vi "(SubVI)Scope_Log_Write Header.vi"(8 "에러 입력(에러 없음)":errorcluster, 10 "Scope_Channel Settings":T1[](array[typedef]) {"Address" format="%04x"}, 11 "Path":path) -> (0 "에러 출력":errorcluster, 3 "File Ref":refnum<file>)   [LabVIEW 2020]
uses:
  Controls/(Ctrl)Scope_Settings.ctl
  e063a442-55f0-4c5f-88aa-a2279cc821e3.vi
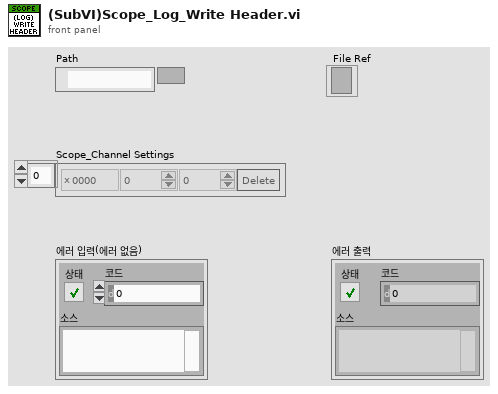
[diagram p1: front panel]
types:
  T1 = typedef "(Ctrl)Scope_Settings.ctl" = cluster{"Address":u16, "Scale":i32, "Offset":i32, "Delete":bool}
  T2 = enum16{"open", "replace", "create", "open or create", "replace or create", "replace or create with confirmation"}
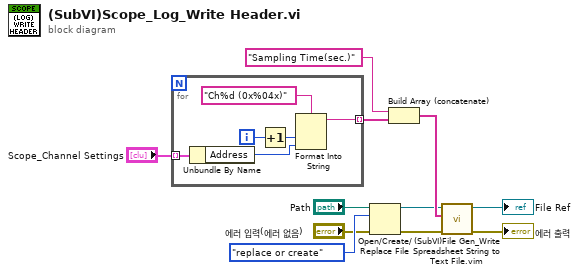
[diagram p0: block diagram]
diagram:
  n1 = for {
    tunnel: "Scope_Channel Settings" -> [w17] mode=indexing
    tunnel: [w12] -> w5 mode=indexing
    i -> [w16]
    n2 = Unbundle By Name(w17) -> ("Address"=w13:u16)
    n3 = Increment(x=w16) -> (x+1=w14:i32)
    n4 = Format Into String(format string="Ch%d (0x%04x)" ("포맷 문자열"), w14, w13) -> (resulting string=w12:string)  [unwired: 2 in, 1 out]
  }
  n5 = Open/Create/Replace File(file path (use dialog)="Path", error in="에러 입력(에러 없음)", operation (0:open)=T2."replace or create" ("동작(0:open)")) -> (refnum out=w7:refnum<file>, error out=w8:errorcluster)  [unwired: 3 in, 1 out]
  n6 = Build Array (concatenate)("Sampling Time(sec.)" ("배열"), w5) -> (w11:string[])
  n7 = call "(SubVI)File Gen_Write Spreadsheet String to Text File.vim"("Error In"=w8, "Array"=w11, "File Ref In"=w7) -> ("Error Out"=→"에러 출력":errorcluster, "File Ref Out"=→"File Ref":refnum<file>)  [unwired: 7 in]
